vi "FGA Get Active Waypoint.vi"() -> (0 "LocalWaypointRec":T1, 1 "ElementUID":u16)   [LabVIEW 2009]
uses:
  LocalWaypointRec.ctl
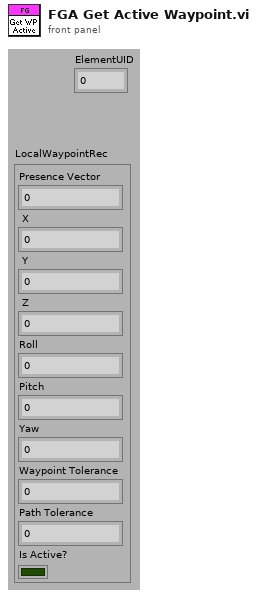
[diagram p1: front panel]
types:
  T1 = typedef "LocalWaypointRec.ctl" = cluster{"Presence Vector":u8, " X":dbl, " Y":dbl, " Z":dbl, "Roll":dbl, "Pitch":dbl, "Yaw":dbl, "Waypoint Tolerance":dbl, "Path Tolerance":dbl, "Is Active?":bool}
  T2 = typedef "ElementRec.ctl" = cluster{"ElementUID":u16, " PreviousUID":u16, " NextUID":u16, "LocalWaypointRec":T1}
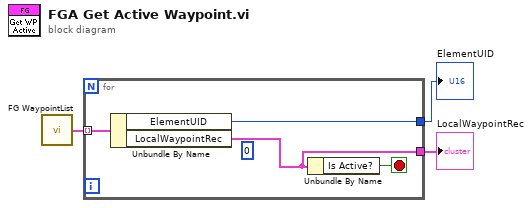
[diagram p0: block diagram]
diagram:
  n1 = call "FG WaypointList.vi"() -> ("Local Waypoint List out"=w2:T2[])  [unwired: 2 in]
  n2 = for {
    tunnel: [w4] -> w3
    tunnel: w2 -> [w7] mode=indexing
    tunnel: [w6] -> w1
    stop <- w5 stop-if-true
    (unwired) 0 ("index")
    n3 = Unbundle By Name(w7) -> ("ElementUID"=w6:u16, "LocalWaypointRec"=w4:T1)
    n4 = Unbundle By Name(w4) -> ("Is Active?"=w5:bool)
  }
  "ElementUID" <- w1
  "LocalWaypointRec" <- w3
